vi "Remove duplicate indices.vi"(1 "I32 array with duplicates":i32[](array[numeric])) -> (0 "I32 array without duplicates":i32[](array[numeric]))   [LabVIEW 2014]
panel:
  # "PN 18/01/2015"
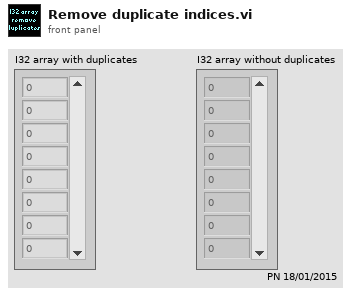
[diagram p1: front panel]
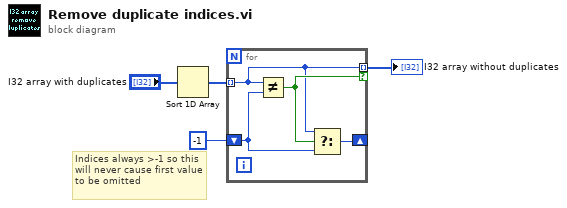
[diagram p0: block diagram]
diagram:
  # "Indices always >-1 so this will never cause first value to be omitted"
  n1 = Sort 1D Array(array="I32 array with duplicates") -> (sorted array=w3:i32[])
  n2 = for {
    tunnel: w3 -> [w6] mode=indexing
    shift-right: [w8] -> _
    shift-left: -1 -> [w5]
    tunnel: [w6] -> w1 mode=indexing if=w7
    n3 = Not Equal?(x=w6, y=w5) -> (x != y?=w7:bool)
    n4 = Select(t=w6, s=w7, f=w5) -> (s? t:f=w8:i32)
  }
  "I32 array without duplicates" <- w1
